vi "Current Y Value Read.vi"(4 "error in (no error)":errorcluster, 6 "Container State":T2, 7 "Display State In":T1={"Measure ?"=[], "Direction"=[], "Loop ?"={"Start"=0, "Finish"=2}, "Storage Location"=[], "Show Current Location"=FALSE, "Current Location"=0, "Show y=0"=FALSE, "Program"=[], "Index"=0, "Average During Loop ?"=FALSE, "# of Loops"=1, "Loop Control"={0, 2}, "Units"="", "Digits"=0, "Significant Figures (F) or DP (T)"=FALSE, "Rate Mode"=FALSE, "Current Y value"=0.0, "Initial Value"=0.0} {"# of Loops" min=1 step=1; "Index" min=0 step=1; "Program"."Step" min=0.001 max=80.0 step=0.001 format="%.2f"; "Program"."Target" format="%.2f"}) -> (0 "error out":errorcluster, 2 "Value":dbl, 3 "Display State Out":T1={"Measure ?"=[], "Direction"=[], "Loop ?"={"Start"=0, "Finish"=2}, "Storage Location"=[], "Show Current Location"=FALSE, "Current Location"=0, "Show y=0"=FALSE, "Program"=[], "Index"=0, "Average During Loop ?"=FALSE, "# of Loops"=1, "Loop Control"={0, 2}, "Units"="", "Digits"=0, "Significant Figures (F) or DP (T)"=FALSE, "Rate Mode"=FALSE, "Current Y value"=0.0, "Initial Value"=0.0} {"# of Loops" min=1 step=1; "Index" min=0 step=1; "Program"."Step" min=0.001 max=80.0 step=0.001 format="%.2f"; "Program"."Target" format="%.2f"})   [LabVIEW 2012, in "Multi Segment Waveform.xctl"]
uses:
  Multi Segment Waveform.xctl
  <vilib>/_xctls/Container State.ctl
  State.ctl
  <vilib>/_xctls/XControlSupport.lvlib
panel:
  # "Replace the Value Indicator below with an Indicator of desired type.\nDo not remove this Indicator or the others from the connector pane. \nDo not change the connector pane pattern.\nThe Value Indicator should always be the second terminal from top on the output side in the connector pane."
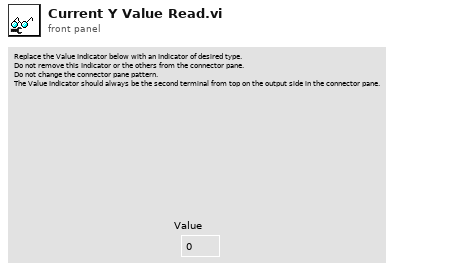
[diagram p1: front panel]
types:
  T1 = typedef "Multi Segment Waveform.xctl/State.ctl" = cluster{"Measure ?":bool[], "Direction":bool[], "Loop ?":cluster{"Start":i32, "Finish":i32}, "Storage Location":i32[], "Show Current Location":bool, "Current Location":i32, "Show y=0":bool, "Program":cluster{"Target":dbl, "Step":dbl, "Measure ?":bool}[], "Index":i32, "Average During Loop ?":bool, "# of Loops":u32, "Loop Control":cluster{i32, i32}, "Units":string, "Digits":i32, "Significant Figures (F) or DP (T)":bool, "Rate Mode":bool, "Current Y value":dbl, "Initial Value":dbl}
  T2 = typedef "XControlSupport.lvlib/Container State.ctl" = cluster{"Indicator?":bool, "Run Mode?":bool, " Refnum":refnum<vi>}
  T3 = cluster{"Target":dbl, "Step":dbl, "Measure ?":bool}[]
  T4 = typedef "Multi Segment Waveform.xctl/Data.ctl" = waveform(dbl)
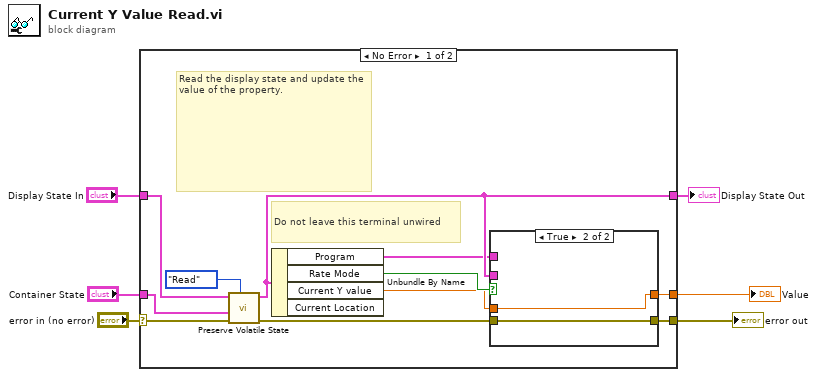
[diagram p0: block diagram]
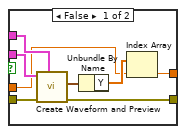
[diagram p2: hidden frame]
diagram:
  n1 = case shown="No Error" "error in (no error)" {
    selector: "error in (no error)" -> [w16 w29]
    tunnel: "Display State In" -> [w17 w28]
    tunnel: [w13 w28] -> w2
    tunnel: "Container State" -> [w15 _]
    tunnel: [w10 w29] -> w1
    tunnel: [w7 _] -> w3
    frame No Error {
      # "Do not leave this terminal unwired"
      # "Read the display state and update the value of the property."
      n2 = call "Preserve Volatile State.vi"("Operation"=enum16{"Read", "Write"}."Read", "error in (no error)"=w16, "Container State"=w15, "Waveform State In"=w17) -> ("error out"=w11:errorcluster, "Waveform State Out"=w13:T1)  [unwired: 1 in, 5 out]
      n3 = Unbundle By Name(w13) -> ("Program"=w12:T3, "Rate Mode"=w9:bool, "Current Y value"=w8:dbl)  [unwired: 1 out]
      n4 = case shown="True" w9 {
        tunnel: w13 -> [w25 _]
        tunnel: w12 -> [w24 _]
        tunnel: w11 -> [w23 w26]
        tunnel: [w22 w26] -> w10
        tunnel: w8 -> [w19 w27]
        tunnel: [w18 w27] -> w7
        frame False {
          n5 = call "Create Waveform and Preview.vi"("Program"=w24, "error in (no error)"=w23, "Display State In"=w25) -> ("error out"=w22:errorcluster, "Waveform Out"=w21:T4)  [unwired: 4 in, 3 out]
          n6 = Unbundle By Name(w21) -> ("Y"=w20:dbl[])
          n7 = Index Array(array=w20, index=w19) -> (element=w18:dbl)
        }
        frame True {
        }
      }
    }
    frame Error {
    }
  }
  "error out" <- w1
  "Value" <- w3
  "Display State Out" <- w2
